vi "queue.vi"() -> ()   [LabVIEW 2020]
uses:
  <vilib>/Utility/error.llb/DialogType.ctl
panel:
  out "# elements in queue":i32
  in  "Numeric":dbl
  out "Waveform Chart 2":i32(graph)
  out "Waveform Chart":i32(graph)
  in  "stop":bool
  out "x-y*floor(x/y)":i32
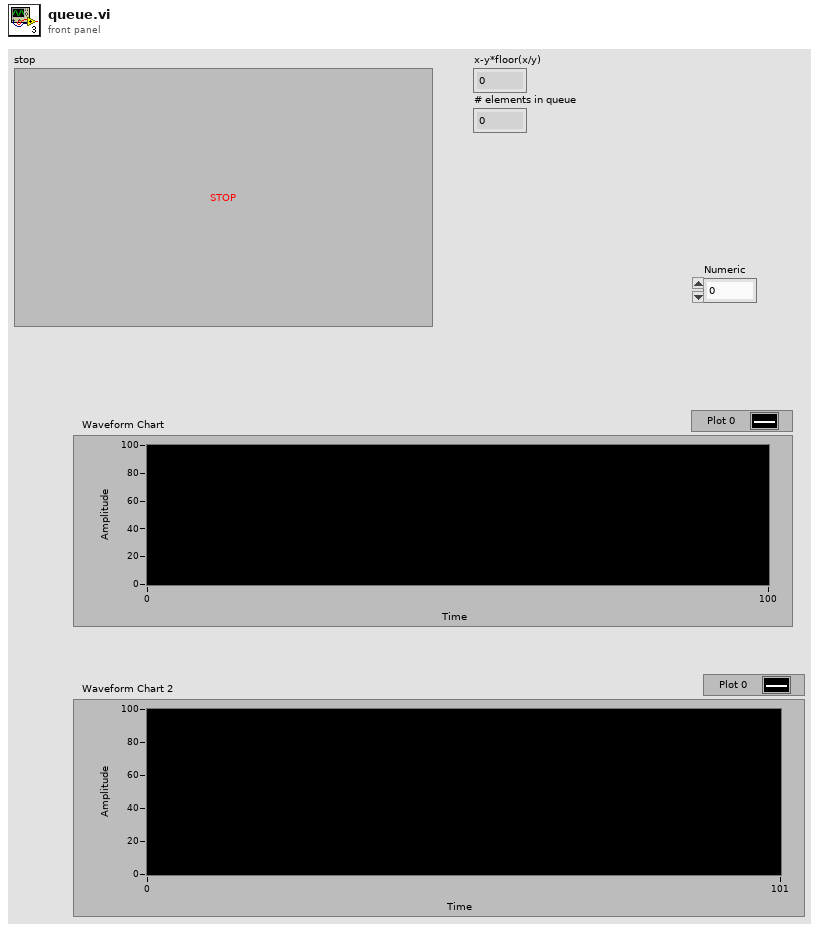
[diagram p1: front panel]
types:
  T1 = typedef "DialogType.ctl" = u16
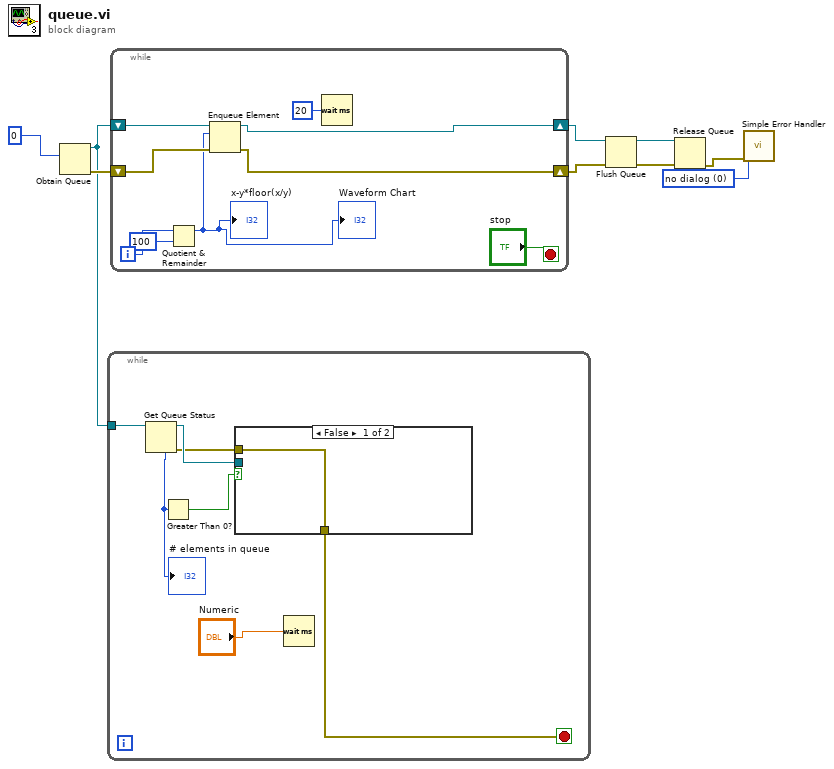
[diagram p0: block diagram]
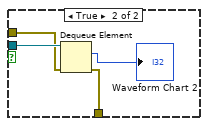
[diagram p2: hidden frame]
diagram:
  w2 = T1 0 items=["no dialog", "OK message", "continue or stop message", "OK message + warnings", "continue/stop + warnings"] ("type of dialog (OK msg:1)")
  n1 = Obtain Queue(element data type=0) -> (queue out=w1:refnum<queue>, error out=w8:errorcluster)  [unwired: 4 in, 1 out]
  n2 = while {
    tunnel: w1 -> [w15]
    stop <- w10 stop-if-true
    n3 = Get Queue Status(queue=w15) -> (queue out=w12:refnum<queue>, error out=w11:errorcluster, # elements in queue=w14:i32)  [unwired: 2 in, 5 out]
    "# elements in queue" <- w14
    n4 = Greater Than 0?(x=w14) -> (x > 0?=w13:bool)
    n5 = case shown="False" w13 {
      tunnel: w12 -> [_ w21]
      tunnel: w11 -> [w17 w20]
      tunnel: [w17 w18] -> w10
      frame False {
      }
      frame True {
        n6 = Dequeue Element(queue=w21, error in (no error)=w20) -> (element=→"Waveform Chart 2":i32, error out=w18:errorcluster)  [unwired: 1 in, 2 out]
      }
    }
    n7 = Wait (ms)(milliseconds to wait="Numeric") -> ()  [unwired: 1 out]
  }
  n8 = while {
    shift-right: [w22] -> w6
    shift-left: w8 -> [w25]
    shift-right: [w23] -> w7
    shift-left: w1 -> [w26]
    i -> [w30]
    stop <- "stop" stop-if-true
    n9 = Quotient & Remainder(x=w30, y=100) -> (x-y*floor(x/y)=w24:i32)  [unwired: 1 out]
    "x-y*floor(x/y)" <- w24
    "Waveform Chart" <- w24
    n10 = Enqueue Element(queue=w26, element=w24, error in (no error)=w25) -> (queue out=w23:refnum<queue>, error out=w22:errorcluster)  [unwired: 1 in, 1 out]
    n11 = Wait (ms)(milliseconds to wait=u32 20) -> ()  [unwired: 1 out]
  }
  n12 = Flush Queue(queue=w7, error in (no error)=w6) -> (queue out=w5:refnum<queue>, error out=w4:errorcluster)  [unwired: 1 out]
  n13 = Release Queue(queue=w5, error in (no error)=w4) -> (error out=w3:errorcluster)  [unwired: 1 in, 2 out]
  n14 = call <vilib>:"Simple Error Handler.vi"("type of dialog (OK msg:1)"=w2, "error in (no error)"=w3) -> ()  [unwired: 3 in, 5 out]
